vi "FTW-Endpoint-Multipart-Tell.vi"(0 "FTW Endpoint":refnum<class "FTW-Endpoint.lvclass">, 5 "Multipart Message":string[](array[string]), 7 "Timeout":i32 format="%dmsec", 11 "error in":errorcluster) -> (4 "FTW Endpoint out":refnum<class "FTW-Endpoint.lvclass">, 6 "Timed out?":bool, 15 "error out":errorcluster)   [LabVIEW 2013, in "FTW-Endpoint.lvclass"]
uses:
  FTW-Endpoint.lvclass
  FTW-Endpoint.lvclass/FTW-Endpoint.ctl
panel:
  # "Inputs"
  # "Outputs"
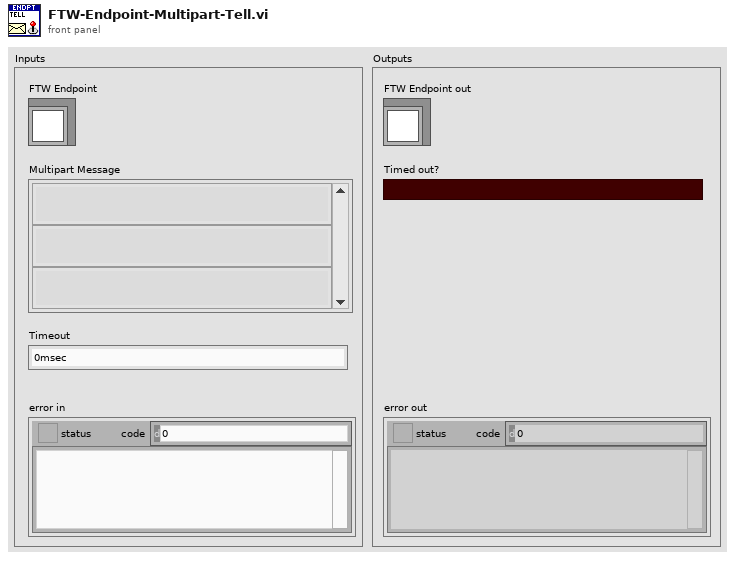
[diagram p1: front panel]
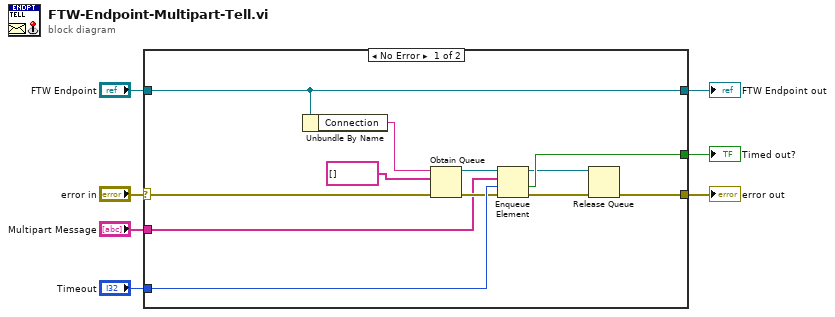
[diagram p0: block diagram]
diagram:
  n1 = case shown="No Error" "error in" {
    selector: "error in" -> [w17 w21]
    tunnel: [w9 w21] -> w7
    tunnel: [w15 w20] -> w5
    tunnel: "FTW Endpoint" -> [w15 w20]
    tunnel: "Multipart Message" -> [w11 _]
    tunnel: [w19 _] -> w2
    tunnel: "Timeout" -> [w18 _]
    frame No Error {
      n2 = Unbundle By Name(w15) -> ("Connection"=w13:string)
      n3 = Obtain Queue(name (unnamed)=w13, element data type=string[] [], error in (no error)=w17) -> (queue out=w12:refnum<queue>, error out=w14:errorcluster)  [unwired: 2 in, 1 out]
      n4 = Enqueue Element(queue=w12, element=w11, timeout in ms (-1)=w18, error in (no error)=w14) -> (queue out=w8:refnum<queue>, timed out?=w19:bool, error out=w16:errorcluster)
      n5 = Release Queue(queue=w8, error in (no error)=w16) -> (error out=w9:errorcluster)  [unwired: 1 in, 2 out]
    }
    frame Error {
    }
  }
  "error out" <- w7
  "FTW Endpoint out" <- w5
  "Timed out?" <- w2
